vi "AWS S3 ls buckets.vi"(8 "error in (no error)":errorcluster, 11 "LV-Data.AWS CLI in":refnum<class "LV-Data.AWS CLI.lvclass">) -> (0 "error out":errorcluster, 2 "Buckets":T1[](array[typedef]), 3 "LV-Data.AWS CLI out":refnum<class "LV-Data.AWS CLI.lvclass">)   [LabVIEW 2019, in "LV-Data.AWS CLI.lvclass"]
uses:
  LV-Data.AWS CLI.lvclass
  Typedefs/AWS CLI.Bucket.ctl
  <vilib>/AWS Toolkit/S3/Bucket/Bucket.lvclass/Bucket.ctl
  LV-Data.S3/LV-Data.S3.lvclass
  <vilib>/AWS Toolkit/S3/Bucket/Bucket.lvclass
panel:
  out "std out":string
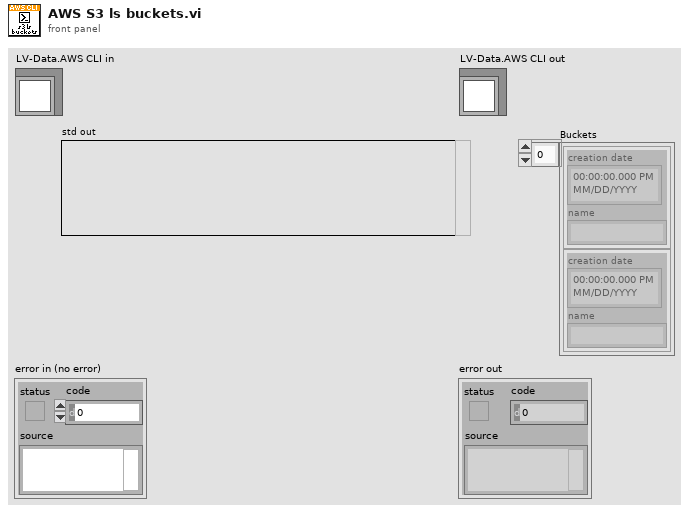
[diagram p1: front panel]
types:
  T1 = typedef "LV-Data.AWS CLI.lvclass/AWS CLI.Bucket.ctl" = cluster{"creation date":timestamp, "name":string}
  T2 = typedef "NI_AWS_Core.lvlib/HTTP Request.lvclass/AWS Credentials.ctl" = cluster{"Access Key":string, "Secret Key":string}
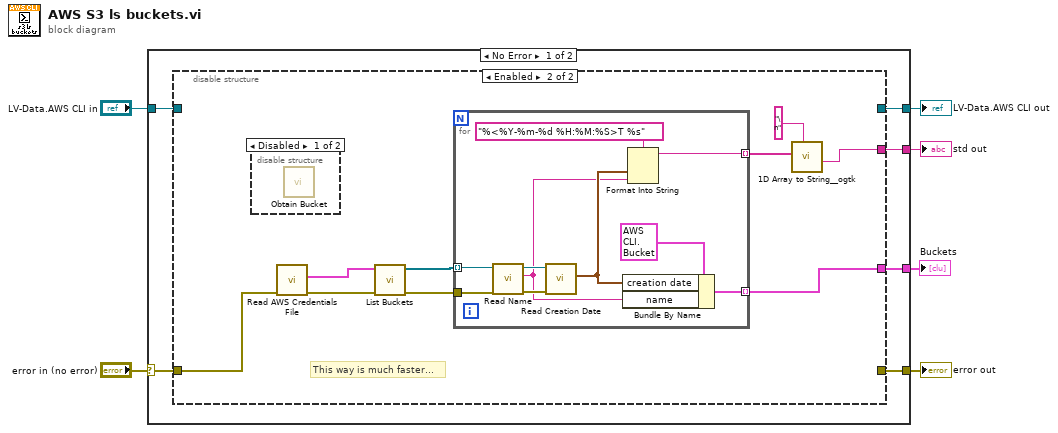
[diagram p0: block diagram]
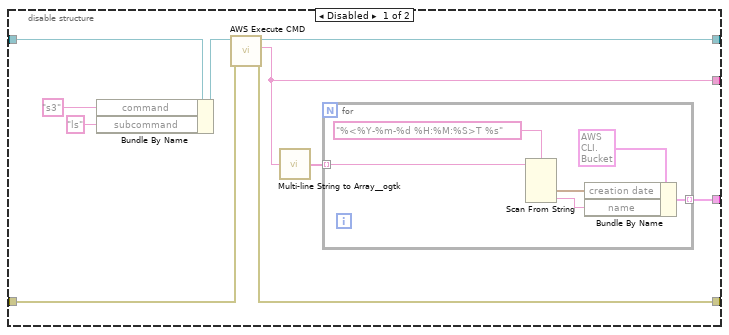
[diagram p2: hidden frame]
diagram:
  n1 = case shown="No Error" "error in (no error)" {
    selector: "error in (no error)" -> [w11 w49]
    tunnel: [w10 w49] -> w5
    tunnel: [w12 w48] -> w3
    tunnel: "LV-Data.AWS CLI in" -> [w9 w48]
    tunnel: [w8 _] -> w2
    tunnel: [w7 _] -> w1
    frame No Error {
      n2 = disable-structure shown="Enabled" {
        disable-tunnel: [w22 _] -> w12
        disable-tunnel: w11 -> [w21 w33]
        disable-tunnel: [w20 _] -> w10
        disable-tunnel: w9 -> [w18 _]
        disable-tunnel: [w15 w29] -> w8
        disable-tunnel: [w13 w32] -> w7
        frame Disabled {
          n3 = Bundle By Name(cluster=w18, "command"="s3" ("CLI.command"), "subcommand"="ls" ("CLI.subcommand")) -> (w19:refnum<class "LV-Data.AWS CLI.lvclass">)
          n4 = call "AWS Execute CMD.vi"("error in (no error)"=w21, "LV-Data.AWS CLI"=w19) -> ("error out"=w20:errorcluster, "std out"=w15:string, "LV-Data.AWS CLI out"=w22:refnum<class "LV-Data.AWS CLI.lvclass">)  [unwired: 7 in]
          n5 = call <userlib>:"Multi-line String to Array__ogtk.vi"("string"=w15) -> ("lines"=w14:string[])
          n6 = for {
            tunnel: w14 -> [w28] mode=indexing
            tunnel: [w24] -> w13 mode=indexing
            n7 = Scan From String(format string="%<%Y-%m-%d %H:%M:%S>T %s", input string=w28) -> (output 1=w26:timestamp, output 2=w23:string)  [unwired: 4 in, 3 out]
            n8 = Bundle By Name(cluster=T1 {"creation date"=timestamp(0 s since 1904-01-01), "name"=""} ("Bucket"), "creation date"=w26, "name"=w23) -> (w24:T1)
          }
        }
        frame Enabled {
          # "This way is much faster..."
          n9 = disable-structure shown="Disabled" {
            frame Disabled {
              n10 = call <vilib>:"Obtain Bucket.vi"() -> ()  [unwired: 10 in, 2 out]
            }
            frame Enabled {
            }
          }
          n11 = call "Read AWS Credentials File.vi"("error in (no error)"=w33) -> ("error out"=w36:errorcluster, "AWS Credentials"=w37:T2)  [unwired: 8 in, 1 out]
          n12 = call <vilib>:"List Buckets.vi"("error in (no error)"=w36, "AWS Credentials"=w37) -> ("error out"=w34:errorcluster, "Buckets"=w35:refnum<class "Bucket.lvclass">[])  [unwired: 6 in, 2 out]
          n13 = for {
            tunnel: w35 -> [w47] mode=indexing
            tunnel: w34 -> [w46]
            tunnel: [w42] -> w32 mode=indexing
            tunnel: [w38] -> w31 mode=indexing
            n14 = call <vilib>:"Read Name.vi"("error in (no error)"=w46, "Bucket in"=w47) -> ("error out"=w43:errorcluster, "Name"=w39:string, "Bucket out"=w44:refnum<class "Bucket.lvclass">)  [unwired: 7 in]
            n15 = call <vilib>:"Read Creation Date.vi"("error in (no error)"=w43, "Bucket in"=w44) -> ("Creation Date"=w41:timestamp)  [unwired: 7 in, 2 out]
            n16 = Bundle By Name(cluster=T1 {"creation date"=timestamp(0 s since 1904-01-01), "name"=""} ("Bucket"), "creation date"=w41, "name"=w39) -> (w42:T1)
            n17 = Format Into String(format string="%<%Y-%m-%d %H:%M:%S>T %s", w41, w39) -> (resulting string=w38:string)  [unwired: 2 in, 1 out]
          }
          n18 = call <userlib>:"1D Array to String__ogtk.vi"("delimiter (Tab)"="\n", "Array of Strings"=w31) -> ("delimited string"=w29:string)  [unwired: 9 in]
        }
      }
    }
    frame Error {
    }
  }
  "error out" <- w5
  "LV-Data.AWS CLI out" <- w3
  "std out" <- w2
  "Buckets" <- w1
